vi "Send Launch Nested Actors.vi"(7 "Message Priority (Normal)":T2=enum."Normal", 8 "error in (no error)":errorcluster, 10 "Nested Actors":T1, 11 "Message Enqueuer":refnum<class "Message Enqueuer.lvclass">) -> (0 "error out":errorcluster, 3 "Message Enqueuer out":refnum<class "Message Enqueuer.lvclass">)   [LabVIEW 2016, in "LHW-GUI.lvlib" / "Launch Nested Actors Msg.lvclass"]
doc: "This VI sends the message to an actor."
uses:
  Launch Nested Actors Msg.lvclass
  <vilib>/ActorFramework/Message Enqueuer/Message Enqueuer.lvclass
  <vilib>/ActorFramework/Message Enqueuer/Message Priority.ctl
  LHW-Acquisition/LHW-Aquisition-Actor.lvclass
  LHW-Analysis/LHW-Analysis-Actor.lvclass
  LHW-Storage/LHW-Storage-Actor.lvclass
  C:/Program Files (x86)/National Instruments/LabVIEW 2016/vi.lib/ActorFramework/Message/Message.lvclass
  Launch Nested Actors Msg.lvclass/Launch Nested Actors Msg.ctl
  <vilib>/ActorFramework/Message Enqueuer/Message Enqueuer.lvclass/Message Enqueuer.ctl
  <vilib>/ActorFramework/Message Priority Queue/Priority Enqueue.vi
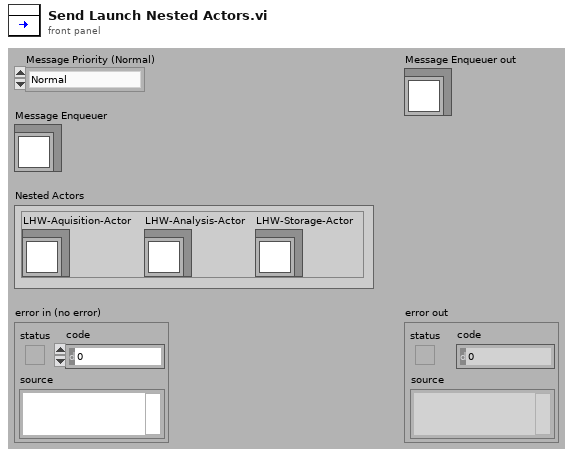
[diagram p1: front panel]
types:
  T1 = cluster{"LHW-Aquisition-Actor":refnum<class "LHW-Aquisition-Actor.lvclass">, "LHW-Analysis-Actor":refnum<class "LHW-Analysis-Actor.lvclass">, "LHW-Storage-Actor":refnum<class "LHW-Storage-Actor.lvclass">}
  T2 = typedef "Actor Framework.lvlib/Message Enqueuer.lvclass/Message Priority.ctl" = enum16{"Low", "Normal", "High"}
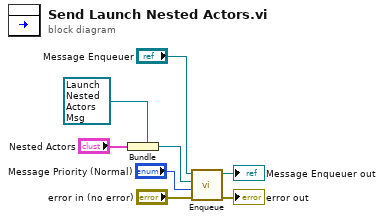
[diagram p0: block diagram]
diagram:
  n1 = Bundle(cluster=refnum<class "Launch Nested Actors Msg.lvclass"> refnum ("Object"), "Nested Actors") -> (w4:refnum<class "Launch Nested Actors Msg.lvclass">)
  n2 = call <vilib>:"Enqueue.vi"("error in (no error)"="error in (no error)", "Message Priority (Normal)"="Message Priority (Normal)", "Message"=w4, "Message Enqueuer in"="Message Enqueuer") -> ("error out"=→"error out":errorcluster, "Message Enqueuer out"=→"Message Enqueuer out":refnum<class "Message Enqueuer.lvclass">)  [unwired: 6 in]
